vi "RT_RW_1ADC_W_DACs.vi"() -> ()   [LabVIEW 2018]
uses:
  <vilib>/FPGAPlugInAG/myRIO-1900/niLvFpga_Open_myRIO-1900.vi
  <vilib>/rvi/interface/common/dynamic/niFpgaDynamicAddResources.vi
  <vilib>/Utility/error.llb/Error Cluster From Error Code.vi
  <vilib>/rvi/errors/niLvFpgaAdjustHostInterfaceError.vi
  <vilib>/FPGAPlugInAG/Dynamic/niLvFpga_Close_Dynamic.vi
  <vilib>/rvi/interface/nirviOpenFPGA/nirviOpenFPGA.xnode
  FPGA Bitfiles/ASPE2019amplifie_FPGATarget_fpgaW&RADCsW3DAC_wVmMEUup6F8.lvbitx
  <vilib>/rvi/interface/nirviReadWriteControl/nirviReadWriteControl.xnode
  <vilib>/rvi/interface/nirviCloseFPGA/nirviCloseFPGA.xnode
  NiFpgaLv.dll
  <vilib>/rvi/interface/Simulation/niFpgaSimulationCallBeginRW.vi
panel:
  in  "ADC 1 write":bool[](array[boolean])=[FALSE, FALSE, FALSE, FALSE, FALSE, TRUE, FALSE, FALSE, FALSE, FALSE, FALSE, FALSE, FALSE, FALSE, FALSE, FALSE]
  out "loop rate (kHz)":dbl
  in  "DAC (V)":dbl
  in  "Stop Button":bool
  out "CH1 (V)":dbl(graph)=-0.3778018523887268
  # "one can enter the voltage input here to actuate a voice coil"
  # "Above is the configured to read +/-10 V range in differential modeusing CH1 of ADC"
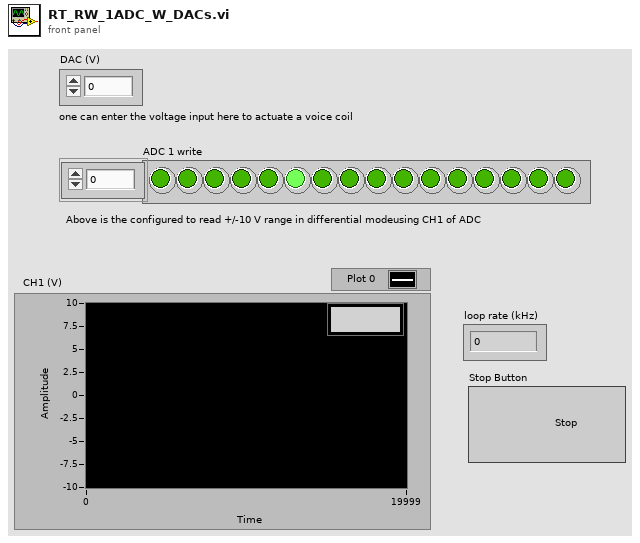
[diagram p1: front panel]
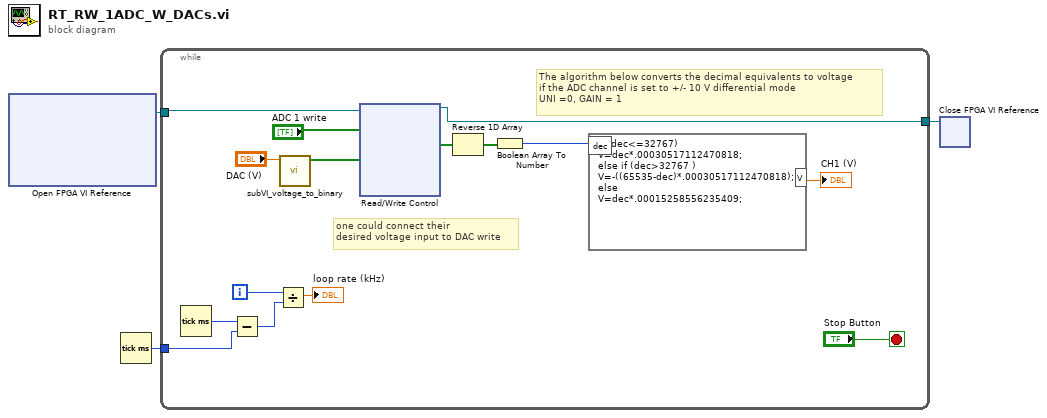
[diagram p0: block diagram]
diagram:
  n1 = xnode "Open FPGA VI Reference"() -> ("FPGA VI Reference Out"=w3:refnum<k20>)  [unwired: 2 in, 1 out]
  n2 = Tick Count (ms)() -> (millisecond timer value=w2:u32)
  n3 = while {
    tunnel: w3 -> [w18]
    tunnel: w2 -> [w13]
    tunnel: [w4] -> w1
    i -> [w12]
    stop <- "Stop Button" stop-if-true
    # "one could connect their \ndesired voltage input to DAC write"
    # "The algorithm below converts the decimal equivalents to voltage\nif the ADC channel is set to +/- 10 V differential mode\nUNI =0, GAIN = 1"
    n4 = Tick Count (ms)() -> (millisecond timer value=w14:u32)
    n5 = Subtract(x=w14, y=w13) -> (x-y=w11:u32)
    n6 = Divide(x=w12, y=w11) -> (x/y=→"loop rate (kHz)":dbl)
    n7 = call "subVI_voltage_to_binary.vi"("voltage"="DAC (V)") -> ("binary"=w7:bool[])  [unwired: 10 in]
    n8 = xnode "Read/Write Control"("FPGA VI Reference In"=w18, "ADC write"="ADC 1 write", "DAC 1 write"=w7) -> ("FPGA VI Reference Out"=w4:refnum<k20>, "ADC read"=w15:bool[])  [unwired: 3 in, 1 out]
    n9 = Reverse 1D Array(array=w15) -> (reversed array=w16:bool[])
    n10 = Boolean Array To Number(Boolean array=w16) -> (number=w9:u16)
    n11 = formula code="if (dec<=32767)\nV=dec*.00030517112470818;\nelse if (dec>32767 )\nV=-((65535-dec)*.00030517112470818);\nelse\nV=dec*.00015258556235409;"("dec"=w9) -> ("V"=→"CH1 (V)":dbl)
  }
  n12 = xnode "Close FPGA VI Reference"("FPGA VI Reference In"=w1) -> ()  [unwired: 1 in, 1 out]
